vi "API_GetCurrentDirectory.vi"() -> (0 "Directory":path)   [LabVIEW 2011, in "API.lvlib"]
uses:
  API.lvlib
  kernel32.dll
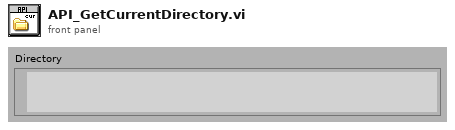
[diagram p1: front panel]
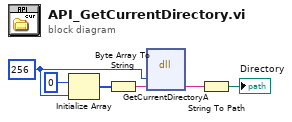
[diagram p0: block diagram]
diagram:
  w6 = 256 ("dimension size")
  n1 = Initialize Array(u8 0 ("element"), w6) -> (w4:u8[])
  n2 = Byte Array To String(unsigned byte array=w4) -> (string=w3:string)
  n3 = dll-call lib="kernel32.dll" fn="GetCurrentDirectoryA" label="GetCurrentDirectory"("nBufferLength"=w6, "Directory"=w3) -> ("Directory"=w2:string)  [unwired: 5 in, 2 out]
  n4 = String To Path(string=w2) -> (path=→"Directory":path)
